vi "temp1.vi"() -> ()   [LabVIEW 2015]
uses:
  timing_tools/poly_asynch_wait_start.vi
  timing_tools/_timing_tools_polys.lvlib
  timing_tools/poly_asynch_wait_wait.vi
panel:
  in  "stop":bool
  out "error out 2":errorcluster
  out "error out":errorcluster
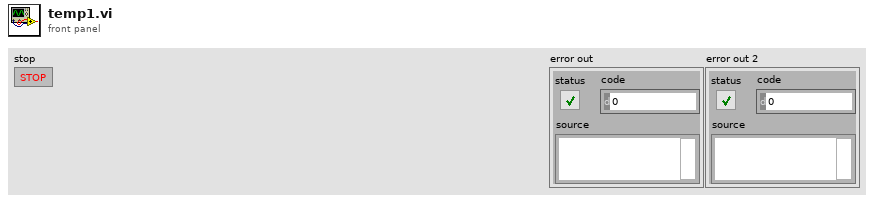
[diagram p1: front panel]
types:
  T1 = typedef "_timing_tools_polys.lvlib/asynch_wait_ref.ctl" = cluster{"vi ref":refnum<vi>, "occ":refnum<k4>}
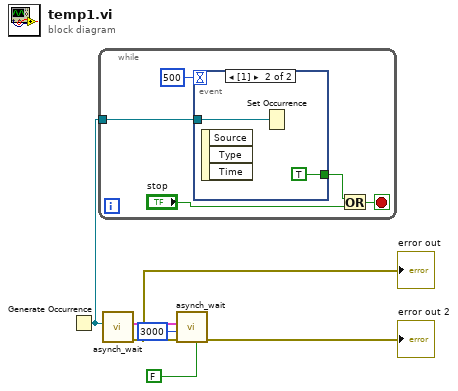
[diagram p0: block diagram]
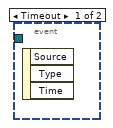
[diagram p2: hidden frame]
diagram:
  n1 = Generate Occurrence() -> (w3:refnum<k4>)
  n2 = while {
    tunnel: w3 -> [w11]
    stop <- w7 stop-if-true
    n3 = event shown="[1]" {
      selector: _ -> [_ _]
      dyn-events: _ -> [_ _]
      timeout: 500 -> [_ _]
      tunnel: w11 -> [_ w13]
      tunnel: [_ TRUE] -> w9
      event Timeout {
        n4 = event-data() -> ()  [unwired: 1 in, 3 out]
      }
      event #1 (no event record) {
        n5 = event-data() -> ()  [unwired: 1 in, 3 out]
        n6 = Set Occurrence(w13) -> ()
      }
    }
    n7 = Or(x=w9, y="stop") -> (x .or. y?=w7:bool)
  }
  n8 = call-poly "asynch_wait.vi"("occ (create)"=w3) -> ("error out"=w6:errorcluster, "asynch wait ref out"=w5:T1)  [unwired: 8 in, 1 out]
  "error out" <- w6
  n9 = call-poly "asynch_wait.vi"("restart asynch wait?"=FALSE, "error in"=w6, "timeout [ms]"=3000, "asynch wait ref in"=w5) -> ("error out"=→"error out 2":errorcluster)  [unwired: 5 in, 2 out]
